vi "Write Button.vi"(6 "Button":u16, 11 "Handle Drag Starting Msg in":refnum<class "Handle Drag Starting Msg.lvclass">) -> (3 "Handle Drag Starting Msg out":refnum<class "Handle Drag Starting Msg.lvclass">)   [LabVIEW 2017, in "File Explorer.lvlib" / "Handle Drag Starting Msg.lvclass"]
uses:
  <vilib>/gpm_packages/@cs/file-explorer-extension/Source/File Explorer/File Explorer Messages/Handle Drag Starting Msg/Handle Drag Starting Msg.lvclass
  <vilib>/gpm_packages/@cs/file-explorer-extension/Source/File Explorer/File Explorer Messages/Handle Drag Starting Msg/Handle Drag Starting Msg.lvclass/Handle Drag Starting Msg.ctl
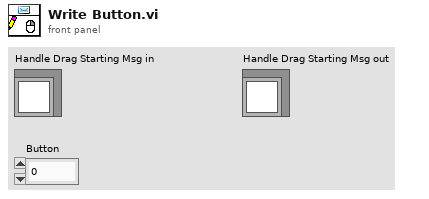
[diagram p1: front panel]
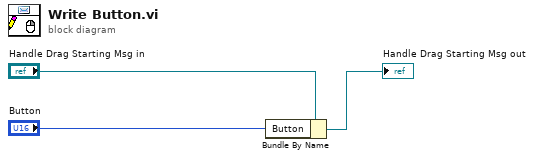
[diagram p0: block diagram]
diagram:
  n1 = Bundle By Name(cluster="Handle Drag Starting Msg in", "Button"="Button") -> (→"Handle Drag Starting Msg out":refnum<class "Handle Drag Starting Msg.lvclass">)
